vi "Instantiate_llm_openai.vi"(0 "model_name":string(combo), 5 "openai_key":string, 11 "error in (no error)":errorcluster) -> (4 "llm_openai out":refnum<class "llm_openai_chatmodels.lvclass">, 15 "error out":errorcluster)   [LabVIEW 2020, in "llm_openai_chatmodels.lvclass"]
uses:
  llm_openai_chatmodels.lvclass
  D:/Personal/LabVIEW LLMs/src/models/abstract_llm_base/abstract_llm_base.lvclass
  llm_openai_chatmodels.lvclass/llm_openai_chatmodels.ctl
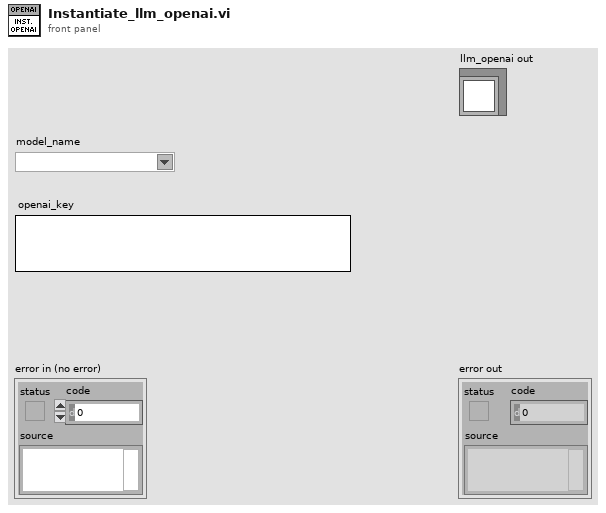
[diagram p1: front panel]
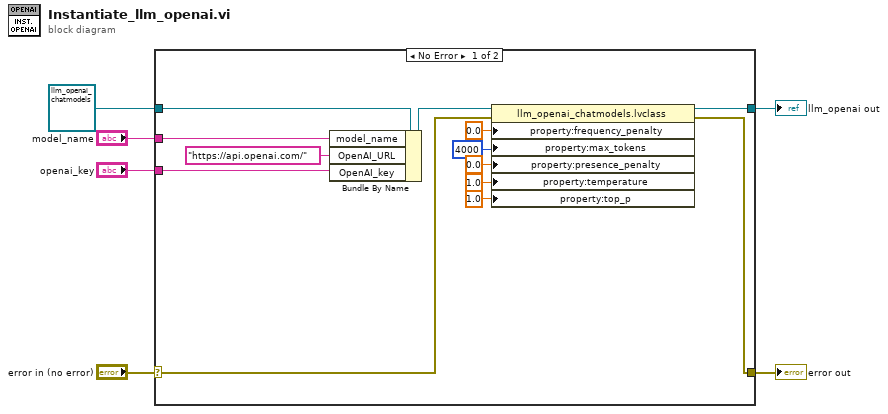
[diagram p0: block diagram]
diagram:
  n1 = case shown="No Error" "error in (no error)" {
    selector: "error in (no error)" -> [w13 w21]
    tunnel: [w12 w21] -> w5
    tunnel: [w14 w20] -> w3
    tunnel: refnum<class "llm_openai_chatmodels.lvclass"> refnum ("llm_openai in") -> [w19 w20]
    tunnel: "model_name" -> [w18 _]
    tunnel: "openai_key" -> [w16 _]
    frame No Error {
      n2 = Bundle By Name(cluster=w19, "model_name"=w18, "OpenAI_URL"="https://api.openai.com/", "OpenAI_key"=w16) -> (w15:refnum<class "llm_openai_chatmodels.lvclass">)
      n3 = property class="llm_openai_chatmodels.lvclass"(reference=w15, error in=w13, "property:frequency_penalty"=0.0 ("frequency_penalty"), "property:max_tokens"=u32 4000 ("max_tokens"), "property:presence_penalty"=0.0 ("presence_penalty"), "property:temperature"=1.0 ("temperature"), "property:top_p"=1.0 ("top_p")) -> (reference out=w14:refnum<class "llm_openai_chatmodels.lvclass">, error out=w12:errorcluster)
    }
    frame Error {
    }
  }
  "error out" <- w5
  "llm_openai out" <- w3
